vi "testTwoServersSendCmdStatusToClientsAtSameTime.vi"(8 "error in":errorcluster) -> (0 "error out":errorcluster)   [LabVIEW 2018]
uses:
  <vilib>/addons/_JKI Toolkits/Caraya/classes/Assert/Assert Equal Value_Variant.vi
  src/TcpServer/TcpServer.lvclass
  <vilib>/addons/_JKI Toolkits/Caraya/classes/Test/Test.lvclass
  <vilib>/addons/_JKI Toolkits/Caraya/classes/Assert/Assert.lvclass
panel:
  out "Run Server B error":errorcluster
  out "Run Server A error":errorcluster
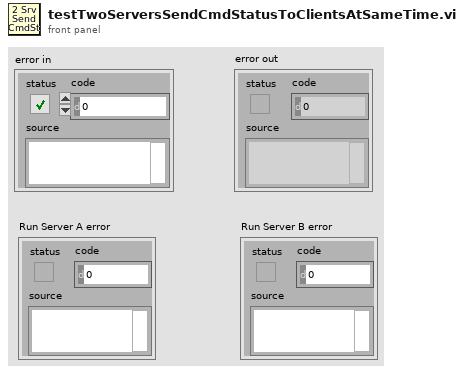
[diagram p1: front panel]
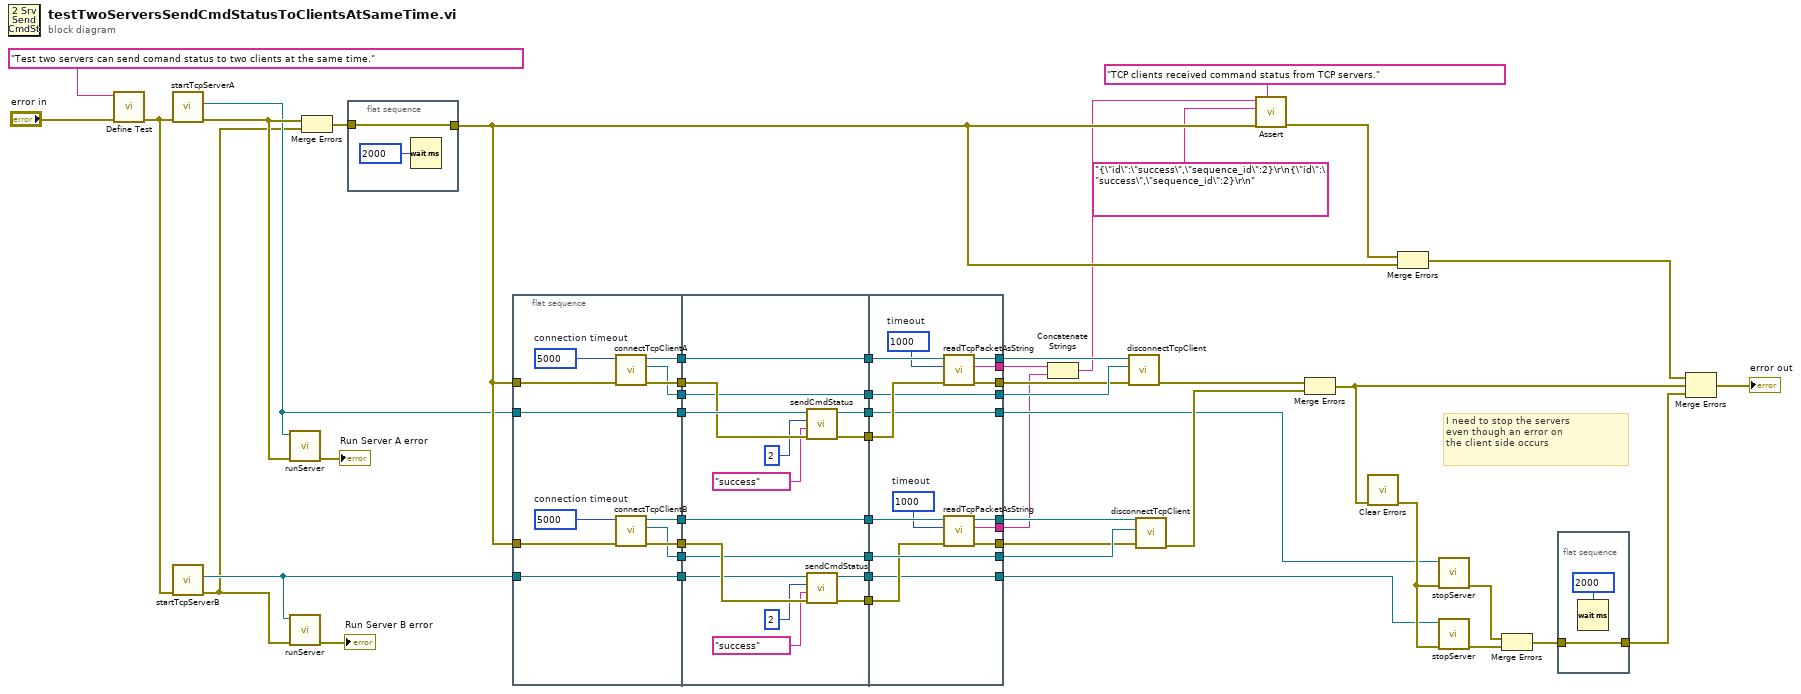
[diagram p0: block diagram]
diagram:
  # "I need to stop the servers \neven though an error on \nthe client side occurs"
  n1 = call <vilib>:"Define Test.vi"("error in (no error)"="error in", "Label (VI Title)"="Test two servers can send comand status to two clients at the same time.") -> ("error out"=w44:errorcluster)  [unwired: 9 in]
  n2 = call "startTcpServerA.vi"("error in (no error)"=w44) -> ("error out"=w39:errorcluster, "TcpServer out"=w35:refnum<class "TcpServer.lvclass">)  [unwired: 8 in, 1 out]
  n3 = call "startTcpServerB.vi"("error in (no error)"=w44) -> ("error out"=w1:errorcluster, "TcpServer out"=w30:refnum<class "TcpServer.lvclass">)  [unwired: 8 in, 1 out]
  n4 = call "runServer.vi"("error in (no error)"=w39, "TcpServer in"=w35) -> ("error out (no error)"=→"Run Server A error":errorcluster)  [unwired: 8 in, 1 out]
  n5 = call "runServer.vi"("error in (no error)"=w1, "TcpServer in"=w30) -> ("error out (no error)"=→"Run Server B error":errorcluster)  [unwired: 8 in, 1 out]
  n6 = Merge Errors(w39, w1) -> (w2:errorcluster)
  n7 = flat-sequence {
    tunnel: [w52] -> w36
    tunnel: w2 -> [w52]
    frame #0 {
      n8 = Wait (ms)(milliseconds to wait=u32 2000) -> ()  [unwired: 1 out]
    }
  }
  n9 = flat-sequence {
    tunnel: w36 -> [w65]
    tunnel: w36 -> [w64]
    tunnel: w35 -> [w63]
    tunnel: [w63] -> w34
    tunnel: [w62] -> w33
    tunnel: [w61] -> w32
    tunnel: [w60] -> w31
    tunnel: w30 -> [w60]
    tunnel: [w59] -> w29
    tunnel: [w58] -> w25
    tunnel: [w57] -> w16
    tunnel: [w56] -> w14
    tunnel: w34 -> [w81]
    tunnel: w33 -> [w80]
    tunnel: w32 -> [w79]
    tunnel: w31 -> [w78]
    tunnel: w29 -> [w77]
    tunnel: [w77] -> w28
    tunnel: [w76] -> w27
    tunnel: w25 -> [w75]
    tunnel: [w75] -> w23
    tunnel: [w74] -> w20
    tunnel: [w71] -> w17
    tunnel: w16 -> [w71]
    tunnel: [w70] -> w15
    tunnel: w14 -> [w70]
    tunnel: [w69] -> w13
    tunnel: [w68] -> w8
    tunnel: w28 -> [w97]
    tunnel: w27 -> [w96]
    tunnel: [w95] -> w26
    tunnel: [w94] -> w24
    tunnel: w23 -> [w94]
    tunnel: [w93] -> w22
    tunnel: [w92] -> w21
    tunnel: w20 -> [w92]
    tunnel: w17 -> [w91]
    tunnel: [w90] -> w11
    tunnel: w15 -> [w90]
    tunnel: w13 -> [w89]
    tunnel: [w88] -> w12
    tunnel: [w87] -> w10
    tunnel: [w86] -> w9
    tunnel: w8 -> [w86]
    tunnel: [w85] -> w5
    tunnel: [w84] -> w6
    frame #0 {
      w54 = 5000  # connection timeout
      w55 = 5000  # connection timeout
      n10 = call "connectTcpClientA.vi"("error in (no error)"=w64, "connection timeout (ms)"=w55) -> ("error out"=w62:errorcluster, "tel connection ID A out"=w58:refnum<k5>, "cmd connection ID A out"=w59:refnum<k5>)  [unwired: 7 in]
      n11 = call "connectTcpClientB.vi"("error in (no error)"=w65, "connection timeout (ms)"=w54) -> ("error out"=w61:errorcluster, "tel connection ID B out"=w56:refnum<k5>, "cmd connection ID B out"=w57:refnum<k5>)  [unwired: 7 in]
    }
    frame #1 {
      n12 = call "sendCmdStatus.vi"("error in (no error)"=w80, "cmdStatus"="success", "sequenceId"=2, "tcpServer in"=w81) -> ("error out"=w76:errorcluster, "tcpServer out"=w74:refnum<class "TcpServer.lvclass">)  [unwired: 6 in]
      n13 = call "sendCmdStatus.vi"("error in (no error)"=w79, "cmdStatus"="success", "sequenceId"=2, "tcpServer in"=w78) -> ("error out"=w69:errorcluster, "tcpServer out"=w68:refnum<class "TcpServer.lvclass">)  [unwired: 6 in]
    }
    frame #2 {
      w82 = 1000  # timeout
      w83 = 1000  # timeout
      n14 = call "readTcpPacketAsString.vi"("error in (no error)"=w96, "timeout ms (1000)"=w83, "connection ID in"=w97) -> ("error out"=w93:errorcluster, "TcpPacket"=w84:string, "connection ID out"=w95:refnum<k5>)  [unwired: 6 in]
      n15 = call "readTcpPacketAsString.vi"("error in (no error)"=w89, "timeout ms (1000)"=w82, "connection ID in"=w91) -> ("error out"=w87:errorcluster, "TcpPacket"=w85:string, "connection ID out"=w88:refnum<k5>)  [unwired: 6 in]
    }
  }
  n16 = Concatenate Strings(w6, w5) -> (w4:string)
  n17 = call "disconnectTcpClient.vi"("error in (no error)"=w22, "tel connection ID in"=w24, "cmd connection ID in"=w26) -> ("error out"=w45:errorcluster)  [unwired: 8 in]
  n18 = call "disconnectTcpClient.vi"("error in (no error)"=w10, "tel connection ID in"=w11, "cmd connection ID in"=w12) -> ("error out"=w43:errorcluster)  [unwired: 8 in]
  n19 = call-poly <vilib>:"Assert.vi"("Label"="TCP clients received command status from TCP servers.", "error in (no error)"=w36, "Y"="{\"id\":\"success\",\"sequence_id\":2}\r\n{\"id\":\"success\",\"sequence_id\":2}\r\n" ("concatenated string"), "X"=w4) -> ("error out"=w38:errorcluster)  [unwired: 7 in]
  n20 = Merge Errors(w45, w43) -> (w41:errorcluster)
  n21 = call <vilib>:"Clear Errors.vi"("error in (no error)"=w41) -> ("error out"=w40:errorcluster)  [unwired: 5 in, 1 out]
  n22 = Merge Errors(w38, w36) -> (w37:errorcluster)
  n23 = call "stopServer.vi"("error in (no error)"=w40, "tcpServer in"=w21) -> ("error out"=w49:errorcluster)  [unwired: 8 in, 1 out]
  n24 = call "stopServer.vi"("error in (no error)"=w40, "tcpServer in"=w9) -> ("error out"=w48:errorcluster)  [unwired: 8 in, 1 out]
  n25 = Merge Errors(w49, w48) -> (w47:errorcluster)
  n26 = flat-sequence {
    tunnel: w47 -> [w98]
    tunnel: [w98] -> w42
    frame #0 {
      n27 = Wait (ms)(milliseconds to wait=u32 2000) -> ()  [unwired: 1 out]
    }
  }
  n28 = Merge Errors(w37, w41, w42) -> (→"error out":errorcluster)
